vi "Lin_Rohner_lab1_ex2.vi"() -> ()   [LabVIEW 2019]
uses:
  <vilib>/Platform/TimedLoop/XDataNode/timing_clust.ctl
  <vilib>/Platform/TimedLoop/XDataNode/nitl_modes.ctl
  <vilib>/Platform/TimedLoop/XDataNode/wakeup.ctl
  <vilib>/Analysis/3filter.llb/Filter Passband Type.ctl
  <vilib>/measure/matone.llb/Extract Single Tone Information 1 Chan.vi
  <vilib>/platform/TimedLoop/XDataNode/XDataNode.xnode
  <vilib>/Platform/TimedLoop/XDataNode/XDNodeRunTimeDep.lvlib
  <vilib>/ptbypt/NI_PtbyPt.lvlib
  <vilib>/Analysis/NI_AALBase.lvlib
  <vilib>/measure/NI_MAPro.lvlib
panel:
  out "Combination of the two signals":cluster{"Data":dbl, "Filtered x":dbl}(graph)
  out "filtered amplitude [Acc unit]":dbl
  out "filtered frequency [Hz]":dbl
  out "raw amplitude [Acc unit]":dbl
  out "raw frequency [Hz]":dbl
  out "Filtered Signal":dbl(graph)
  in  "low cutoff freq: fl":dbl=0.125 format="%0.3f"
  in  "Channel select":tag
  out "Raw Signal":dbl(graph)
  in  "READY":bool
  in  "Acceleration in\nm/s^2    or    g":bool
  in  "STOP":bool
  out "Current Sample":dbl
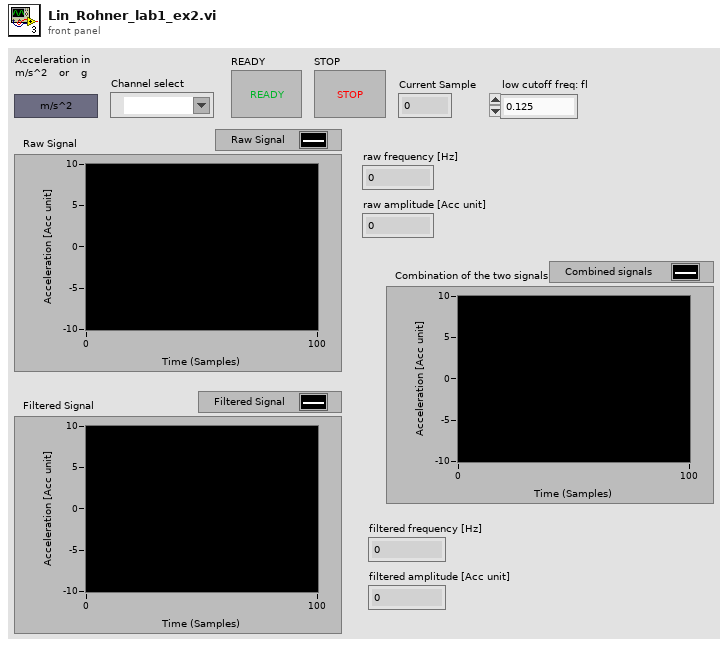
[diagram p1: front panel]
types:
  T1 = typedef "NI_AALBase.lvlib/Filter Passband Type.ctl" = enum32{"Lowpass", "Highpass", "Bandpass", "Bandstop"}
  T2 = typedef "XDNodeRunTimeDep.lvlib/timing_clust.ctl" = cluster{"Expected End [f-1]":u64, "Actual End [f-1]":u64, "Finished Late? [f-1]":bool, "Expected End [i-1]":u64, "Actual End [i-1]":u64, "Finished Late? [i-1]":bool, "Expected Start [i]":u64, "Actual Start [i]":u64, "Expected Start [f]":u64, "Actual Start [f]":u64, "Source Name":string, "Structure Name":string, "Period":i64, "Deadline":i64, "Offset":i64, "Start":i64, "Priority":i32, "Timeout":i32, "Mode":T3, "Wakeup Reason":T4, "Error":errorcluster, "Source Type":string, "Secondary Source Type":string, "Global End Time":u64, "Global Start Time":u64, "Frame Duration":u64, "Iteration Duration":u64, "Assigned CPU":i32, "I/O Scan Engine Mode":u32}
  T3 = typedef "XDNodeRunTimeDep.lvlib/nitl_modes.ctl" = enum32{"No Change", "Process missed periods, maintain original phase", "Discard missed periods, maintain original phase", "Process missed periods, ignore original phase", "Discard missed periods, ignore original phase"}
  T4 = typedef "XDNodeRunTimeDep.lvlib/wakeup.ctl" = enum32{"Normal", "Aborted", "Asynchronous wakeup", "Timing source error", "Timed loop error", "Timeout"}
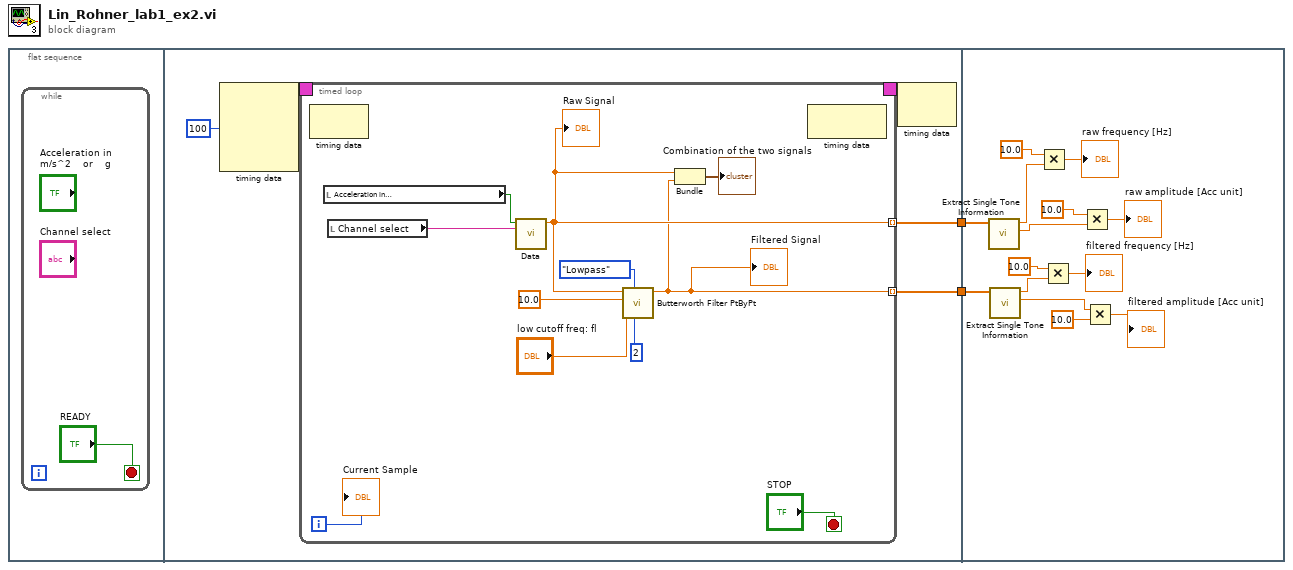
[diagram p0: block diagram]
diagram:
  n1 = flat-sequence {
    tunnel: [w5] -> w2
    tunnel: [w4] -> w1
    tunnel: w2 -> [w39]
    tunnel: w1 -> [w38]
    frame #0 {
      n2 = while {
        stop <- "READY" stop-if-true
      }
    }
    frame #1 {
      n3 = node-c288(i64 100 ("Period")) -> (w8:T2)  [unwired: 3 in]
      n4 = timed-loop {
        timing: w8 -> [_]
        timing-out: [_] -> w7
        tunnel: [w11] -> w5 mode=indexing
        tunnel: [w10] -> w4 mode=indexing
        i -> [w19]
        stop <- "STOP" stop-if-true
        n5 = node-c288() -> ()  [unwired: 1 in, 1 out]
        n6 = local read "Acceleration in\nm/s^2    or    g"() -> (w17:bool)
        n7 = local read "Channel select"() -> (w16:tag)
        n8 = call "Data.vi"("Channel select"=w16, "Acceleration in\nm/s^2    or    g"=w17) -> ("Data"=w11:dbl)  [unwired: 9 in]
        "Raw Signal" <- w11
        n9 = call <vilib>:"Butterworth Filter PtByPt.vi"("order"=2, "filter type"=Filter_Passband_Type."Lowpass", "low cutoff freq: fl"="low cutoff freq: fl", "sampling freq: fs"=10.0, "x"=w11) -> ("Filtered x"=w10:dbl)  [unwired: 4 in, 1 out]
        "Filtered Signal" <- w10
        n10 = Bundle("Data"=w11, "Filtered x"=w10) -> (→"Combination of the two signals":cluster{"Data":dbl, "Filtered x":dbl})  [unwired: 1 in]
        n11 = node-c288() -> ()  [unwired: 1 in, 1 out]
        "Current Sample" <- w19
      }
      n12 = node-c288(w7) -> ()  [unwired: 1 out]
    }
    frame #2 {
      n13 = call-poly <vilib>:"Extract Single Tone Information.vi"("time signal in"=w39) -> ("detected amplitude"=w34:dbl, "detected frequency"=w36:dbl)  [unwired: 5 in, 4 out]
      n14 = call-poly <vilib>:"Extract Single Tone Information.vi"("time signal in"=w38) -> ("detected amplitude"=w31:dbl, "detected frequency"=w37:dbl)  [unwired: 5 in, 4 out]
      n15 = Multiply(x=10.0, y=w36) -> (x*y=→"raw frequency [Hz]":dbl)
      n16 = Multiply(x=10.0, y=w37) -> (x*y=→"filtered frequency [Hz]":dbl)
      n17 = Multiply(x=10.0, y=w34) -> (x*y=→"raw amplitude [Acc unit]":dbl)
      n18 = Multiply(x=w31, y=10.0) -> (x*y=→"filtered amplitude [Acc unit]":dbl)
    }
  }
